vi "Serial_Close.vi"(8 "error in (no error)":errorcluster, 11 "Python in":cluster{"Python":refnum<k35>, "py file":path}) -> ()   [LabVIEW 2020]
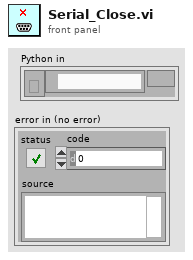
[diagram p1: front panel]
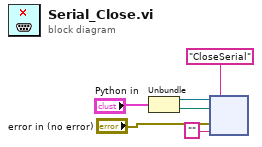
[diagram p0: block diagram]
diagram:
  n1 = Unbundle("Python in") -> ("Python"=w1:refnum<k35>, "py file"=w6:path)
  n2 = node(w1, w6, "CloseSerial" ("function name"), "error in (no error)", "" ("function name")) -> ()  [unwired: 1 in, 4 out]
